vi "Validate Transmit SubAddresses.vi"(6 "RT 1?":bool, 8 "error in (no error)":errorcluster, 11 "RT Config in":refnum<class "RT Config.lvclass">) -> (0 "error out":errorcluster, 3 "RT Config out":refnum<class "RT Config.lvclass">)   [LabVIEW 2016, in "RT Config.lvclass"]
uses:
  RT Config.lvclass
  PPLs/FPGA Interface.lvlibp/FPGA Interface/FPGA Interface.lvclass
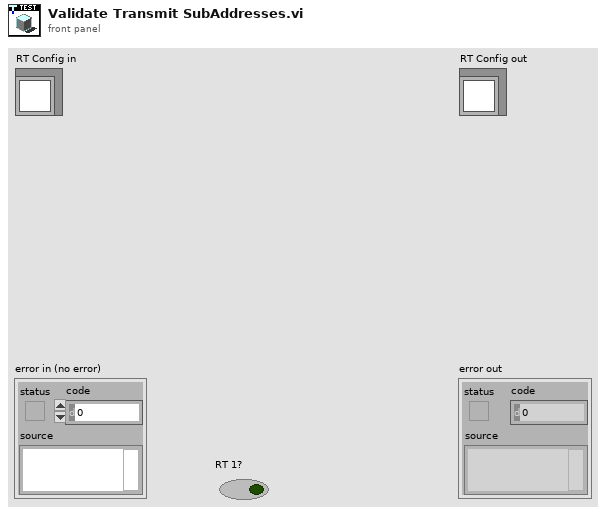
[diagram p1: front panel]
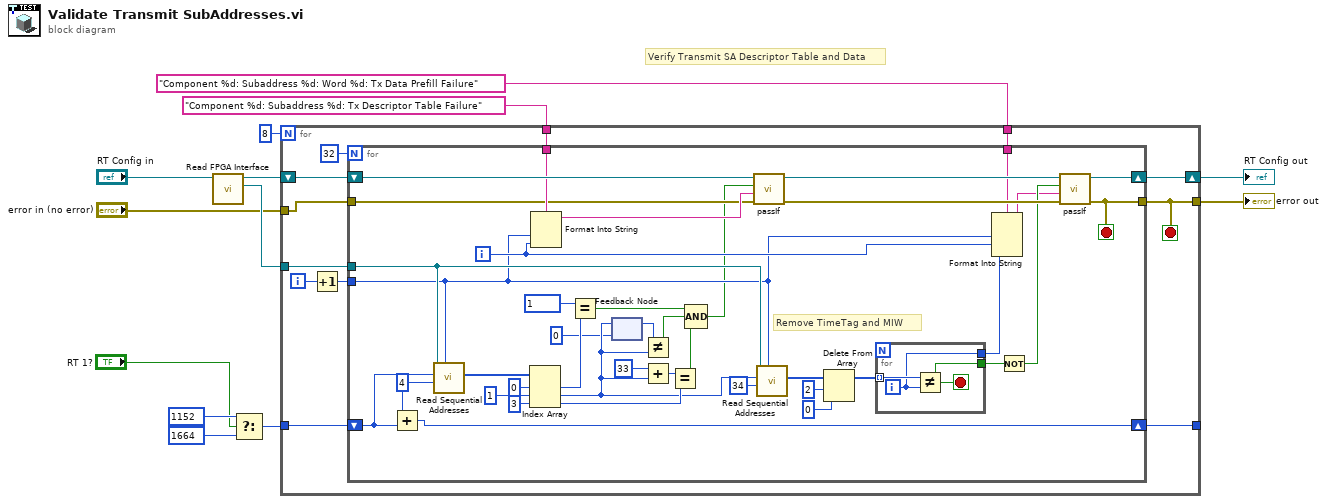
[diagram p0: block diagram]
diagram:
  # "Verify Transmit SA Descriptor Table and Data"
  n1 = call-dynamic "Read FPGA Interface.vi"("1553 Test in"="RT Config in") -> ("FPGA Interface"=w12:refnum<class "FPGA Interface.lvclass">, "1553 Test out"=w7:refnum<class "RT Config.lvclass">)  [unwired: 8 in, 1 out]
  n2 = Select(t=u16 1152, s="RT 1?", f=u16 1664) -> (s? t:f=w8:u16)
  n3 = for {
    N: 8 -> [_]
    tunnel: w12 -> [w22]
    shift-right: [w19] -> w5
    shift-left: w7 -> [w20]
    tunnel: "Component %d: Subaddress %d: Tx Descriptor Table Failure" ("message (\"\")") -> [w18]
    tunnel: w8 -> [w24]
    tunnel: [w23] -> _
    tunnel: [w16] -> w4
    tunnel: "error in (no error)" -> [w15]
    tunnel: "Component %d: Subaddress %d: Word %d: Tx Data Prefill Failure" ("message (\"\")") -> [w14]
    i -> [w25]
    stop <- w16 stop-if-true
    n4 = Increment(x=w25) -> (x+1=w21:i32)
    n5 = for {
      N: 32 -> [_]
      tunnel: w22 -> [w58]
      tunnel: w21 -> [w43]
      tunnel: w18 -> [w56]
      shift-right: [w63] -> w23
      shift-left: w24 -> [w64]
      shift-right: [w50] -> w19
      shift-left: w20 -> [w57]
      tunnel: [w48] -> w16
      tunnel: w15 -> [w47]
      tunnel: w14 -> [w46]
      i -> [w44]
      stop <- w48 stop-if-true
      w65 = u16 4 ("Addresses to Read")
      # "Remove TimeTag and MIW"
      n6 = Add(x=w65, y=w64) -> (x+y=w63:u16)
      n7 = call-dynamic "Read Sequential Addresses.vi"("Target IC (1-8)"=w43, "Addresses to Read"=w65, "Starting Address"=w64, "FPGA Interface in"=w58) -> ("Data"=w62:u16[])  [unwired: 6 in, 1 out]
      n8 = Index Array(array=w62, index #1=0 ("index"), index #2=1 ("index"), index #3=3 ("index")) -> (element #1=w35:u16, element #2=w30:u16, element #3=w31:u16)
      n9 = Format Into String(format string=w56, w43, w44) -> (resulting string=w55:string)  [unwired: 2 in, 1 out]
      n10 = Equal?(x=u16 1, y=w35) -> (x = y?=w38:bool)
      n11 = feedback-in #1(w30) -> ()
      n12 = feedback #1(u16 0 ("Data")) -> (w37:u16)
      n13 = Not Equal?(x=w37, y=w30) -> (x != y?=w36:bool)
      n14 = Add(x=u16 33, y=w30) -> (x+y=w33:u16)
      n15 = Equal?(x=w33, y=w31) -> (x = y?=w32:bool)
      n16 = Compound Arithmetic op=AND(w38, w36, w32) -> (w39:bool)
      n17 = call-dynamic "passIf.vi"("error in (no error)"=w47, "message (\"\")"=w55, "pass"=w39, "TestCase in"=w57) -> ("error out"=w49:errorcluster, "TestCase out"=w51:refnum<class "RT Config.lvclass">)  [unwired: 6 in]
      n18 = call-dynamic "Read Sequential Addresses.vi"("Target IC (1-8)"=w43, "Addresses to Read"=u16 34, "Starting Address"=w30, "FPGA Interface in"=w58) -> ("Data"=w53:u16[])  [unwired: 6 in, 1 out]
      n19 = Delete From Array(array=w53, length=2, index=0) -> (array with subset deleted=w29:u16[])  [unwired: 1 out]
      n20 = for {
        tunnel: w29 -> [w68] mode=indexing
        tunnel: [w67] -> w52
        tunnel: [w66] -> w42
        i -> [w66]
        stop <- w67 stop-if-true
        n21 = Not Equal?(x=w68, y=w66) -> (x != y?=w67:bool)
      }
      n22 = Format Into String(format string=w46, w43, w44, w42) -> (resulting string=w41:string)  [unwired: 2 in, 1 out]
      n23 = Not(x=w52) -> (.not. x?=w45:bool)
      n24 = call-dynamic "passIf.vi"("error in (no error)"=w49, "message (\"\")"=w41, "pass"=w45, "TestCase in"=w51) -> ("error out"=w48:errorcluster, "TestCase out"=w50:refnum<class "RT Config.lvclass">)  [unwired: 6 in]
    }
  }
  "error out" <- w4
  "RT Config out" <- w5
